vi "Main.vi"() -> ()   [LabVIEW 2017]
doc: "The myRIO Project template acquires acceleration data from the onboard accelerometer and displays the changes of acceleration values in a waveform chart."
uses:
  <vilib>/myRIO/Instrument Drivers/Onboard IO/DIO/typedefs/DIO Reference.ctl
  <vilib>/myRIO/Common/Instrument Driver Framework/Utilities/typedefs/myRIO Generic Hardware Reference.ctl
  <vilib>/myRIO/Common/Instrument Driver Framework/Utilities/typedefs/Hardware Version Enum.ctl
  <vilib>/myRIO/Common/Instrument Driver Framework/Utilities/typedefs/myRIO v1.0 Reference.ctl
  <vilib>/myRIO/Common/Instrument Driver Framework/Utilities/typedefs/Generic FPGA Reference.ctl
  <vilib>/myRIO/Common/Instrument Driver Framework/myRIO v1.0/DIO/typedefs/DIO Channels List.ctl
  <vilib>/myRIO/Common/Instrument Driver Framework/myRIO v1.0/DIO/typedefs/DIO Channels Enum.ctl
  <vilib>/userdefined/High Color/nirio_resource_hc.ctl
  <vilib>/Platform/TimedLoop/XDataNode/timing_clust.ctl
  <vilib>/Platform/TimedLoop/XDataNode/nitl_modes.ctl
  <vilib>/Platform/TimedLoop/XDataNode/wakeup.ctl
  <vilib>/myRIO/Instrument Drivers/Onboard IO/PWM/typedefs/PWM Reference.ctl
  <vilib>/myRIO/Common/Instrument Driver Framework/myRIO v1.0/PWM/typedefs/PWM Channels Enum.ctl
  <vilib>/myRIO/Instrument Drivers/Onboard IO/PWM/typedefs/PWM Configuration.ctl
  <vilib>/myRIO/Common/Instrument Driver Framework/myRIO v1.0/Encoder/typedefs/Encoder Signal Mode.ctl
  <vilib>/myRIO/Instrument Drivers/Onboard IO/Encoder/typedefs/Encoder Reference.ctl
  <vilib>/myRIO/Common/Instrument Driver Framework/myRIO v1.0/Encoder/typedefs/Encoder Channels Enum.ctl
  <vilib>/myRIO/Common/Instrument Driver Framework/myRIO v1.0/Encoder/typedefs/Encoder Configuration v1.0.ctl
  <vilib>/myRIO/Instrument Drivers/Onboard IO/AI/typedefs/AI Reference.ctl
  <vilib>/myRIO/Common/Instrument Driver Framework/myRIO v1.0/AI/typedefs/AI Channels List.ctl
  <vilib>/myRIO/Common/Instrument Driver Framework/myRIO v1.0/AI/typedefs/AI Channels Enum.ctl
  <vilib>/myRIO/Common/Instrument Driver Framework/Utilities/typedefs/Analog Scaling Constants List.ctl
  <vilib>/myRIO/Common/Instrument Driver Framework/Utilities/typedefs/Analog Scaling Constants.ctl
  <vilib>/myRIO/Common/Instrument Driver Framework/Utilities/vis/Is FPGA Ref Available.vi
  <vilib>/myRIO/Common/Instrument Driver Framework/myRIO v1.0/DIO/vis/myRIO v1.1 Open DIO.vi
  <vilib>/myRIO/Instrument Drivers/Onboard IO/DIO/vis/Write.vi
  <vilib>/myRIO/Common/Instrument Driver Framework/myRIO v1.0/PWM/vis/myRIO v1.1 Open PWM.vi
  <vilib>/myRIO/Instrument Drivers/Onboard IO/PWM/vis/Set Duty Cycle and Frequency.vi
  <vilib>/myRIO/Common/Instrument Driver Framework/myRIO v1.0/AI/vis/myRIO v1.1 Open AI.vi
  <vilib>/myRIO/Instrument Drivers/Onboard IO/AI/vis/Read.vi
  <vilib>/myRIO/Common/Instrument Driver Framework/myRIO v1.0/Encoder/vis/myRIO v1.1 Open Encoder.vi
  <vilib>/myRIO/Instrument Drivers/Onboard IO/Encoder/vis/Read.vi
  <vilib>/myRIO/Common/Instrument Driver Framework/Utilities/vis/Validate Channels.vi
  <vilib>/myRIO/Common/Instrument Driver Framework/myRIO v1.0/DIO/vis/myRIO v1.0 Reserve DIO.vi
  <vilib>/myRIO/Common/Instrument Driver Framework/myRIO v1.0/PWM/vis/myRIO v1.0 Reserve PWM.vi
  <vilib>/myRIO/Common/Instrument Driver Framework/myRIO v1.0/AI/vis/myRIO v1.0 Reserve AI.vi
  <vilib>/myRIO/Common/Instrument Driver Framework/myRIO v1.0/Encoder/vis/myRIO v1.0 Reserve Encoder.vi
  <vilib>/myRIO/Common/Instrument Driver Framework/myRIO v1.0/Resource Manager/vis/myRIO v1.0 Reserve Channel List.vi
  <vilib>/myRIO/Common/Instrument Driver Framework/myRIO v1.0/DIO/vis/myRIO v1.0 Build MUX Configuration DIO.vi
  <vilib>/myRIO/Common/Instrument Driver Framework/myRIO v1.0/PWM/vis/myRIO v1.0 Build MUX Configuration PWM.vi
  <vilib>/myRIO/Common/Instrument Driver Framework/myRIO v1.0/AI/vis/myRIO v1.0 Build MUX Configuration AI.vi
  <vilib>/myRIO/Common/Instrument Driver Framework/myRIO v1.0/Encoder/vis/myRIO v1.0 Build MUX Configuration Encoder.vi
  <vilib>/myRIO/Common/Instrument Driver Framework/myRIO v1.0/Resource Manager/vis/myRIO v1.0 Reserve Channel.vi
  <vilib>/myRIO/Common/Instrument Driver Framework/myRIO v1.0/Resource Manager/vis/myRIO v1.0 Unreserve Channel.vi
  <vilib>/myRIO/Common/Instrument Driver Framework/myRIO v1.0/Resource Manager/vis/myRIO v1.0 Create Configuration List.vi
  <vilib>/myRIO/Common/Instrument Driver Framework/myRIO v1.0/Resource Manager/vis/myRIO v1.0 Build Mutex Name.vi
  <vilib>/Utility/VariantDataType/GetNumericInfo.vi
  <vilib>/Utility/error.llb/Error Cluster From Error Code.vi
  <vilib>/myRIO/Common/Instrument Driver Framework/myRIO v1.0/myRIO v1.1 Open.vi
  <vilib>/myRIO/Common/Instrument Driver Framework/Utilities/vis/IO Manager.vi
  <vilib>/myRIO/Common/Instrument Driver Framework/Utilities/vis/Configuration Manager.vi
  <vilib>/myRIO/Common/Instrument Driver Framework/myRIO v1.0/Resource Manager/vis/myRIO v1.0 Configure IO.vi
  <vilib>/myRIO/Common/Instrument Driver Framework/myRIO v1.0/myRIO v1.0 Close.vi
  <vilib>/myRIO/Common/Instrument Driver Framework/myRIO v1.0/DIO/vis/myRIO v1.0 Write DIO.vi
  <vilib>/myRIO/Common/Instrument Driver Framework/myRIO v1.0/PWM/vis/myRIO v1.0 Write PWM.vi
  <vilib>/myRIO/Common/Instrument Driver Framework/myRIO v1.0/Encoder/vis/myRIO v1.0 Configure Encoder.vi
  <vilib>/myRIO/Common/Instrument Driver Framework/myRIO v1.0/Encoder/vis/myRIO v1.0 Read Encoder.vi
  <vilib>/myRIO/Common/Instrument Driver Framework/myRIO v1.0/AI/vis/myRIO v1.0 Get Scaling Constants AI.vi
  <vilib>/myRIO/Common/Instrument Driver Framework/myRIO v1.0/AI/vis/myRIO v1.0 Read AI.vi
  <vilib>/myRIO/Express VI/Onboard IO/DO/DO Express VI.xnode
  <vilib>/myRIO/Instrument Drivers/Onboard IO/DIO/vis/myRIO DIO Open.xnode
  <vilib>/myRIO/Express VI/Onboard IO/PWM/PWM Express VI.xnode
  <vilib>/myRIO/Instrument Drivers/Onboard IO/PWM/vis/myRIO PWM Open.xnode
  <vilib>/platform/TimedLoop/XDataNode/XDataNode.xnode
  <vilib>/myRIO/Express VI/Onboard IO/Encoder/Encoder Express VI.xnode
  <vilib>/myRIO/Instrument Drivers/Onboard IO/Encoder/vis/myRIO Encoder Open.xnode
  <vilib>/myRIO/Express VI/Onboard IO/AI/AI Express VI.xnode
  <vilib>/myRIO/Instrument Drivers/Onboard IO/AI/vis/myRIO AI Open.xnode
  <vilib>/myRIO/Instrument Drivers/Onboard IO/DIO/DIO.lvlib
  <vilib>/myRIO/Instrument Drivers/Onboard IO/PWM/PWM.lvlib
  <vilib>/myRIO/Instrument Drivers/Onboard IO/AI/AI.lvlib
  <vilib>/myRIO/Instrument Drivers/Onboard IO/Encoder/Encoder.lvlib
  <vilib>/Platform/TimedLoop/XDataNode/XDNodeRunTimeDep.lvlib
panel:
  in  "LIMin":dbl=15.0 min=0.0 step=0.1
  out "dt":dbl
  in  "Zerar Rede Neural":bool
  out "Aceleração da Ponta":dbl(graph)
  out "accp":dbl
  out "thpp":dbl
  out "thp":dbl
  out "Thetapp":cluster{"Thetapp":dbl, "thppD":dbl}(graph)
  out "Thetap":cluster{"Thetap":dbl, "thpD":dbl}(graph)
  out "Theta":cluster{"Theta":dbl, "thD":dbl}(graph)
  out "th":dbl
  in  "srpC":dbl=60.0 min=1.0 step=1.0
  in  "kIN":dbl=20.0 min=1.0 step=1.0
  in  "phiIN":dbl=15.0 step=0.1
  in  "apIN":dbl=1.8 min=0.0 step=0.1
  in  "Min":dbl=100.0 min=1.0 step=1.0
  in  "Funcionamento":bool
  in  "Lambda":dbl=15.0 min=0.0 max=10000.0 step=0.1
  in  "Tab Control":T1(tab)=enum."Controle Cossenoidal"
  in  "Posicao Angular":dbl(knob) min=-45.0 max=45.0 step=5.0 scale=45.0..-45.0
  in  "Amplitude":dbl(knob)=45.0 min=0.0 max=45.0 step=1.0 scale=0.0..45.0
  in  "Frequencia (Hz)":dbl(knob)=0.10000000000000002 min=0.0 max=3.0 step=0.1 scale=0.0..3.0
  in  "Amplitude":dbl(knob)=45.0 min=0.0 max=45.0 step=1.0 scale=0.0..45.0
  in  "Frequencia (Hz)":dbl(knob)=0.10000000000000002 min=0.0 max=3.0 step=0.1 scale=0.0..3.0
  in  "Período":dbl(knob)=2.5 min=1.5 max=10.0 step=0.5 scale=1.5..10.0
  in  "Reducao de vibração":bool=TRUE
  in  "Ciclo de Controle":bool
  out "th(°)":dbl
  in  "Zerar contador":bool
  in  "Ciclo de aquisição":bool
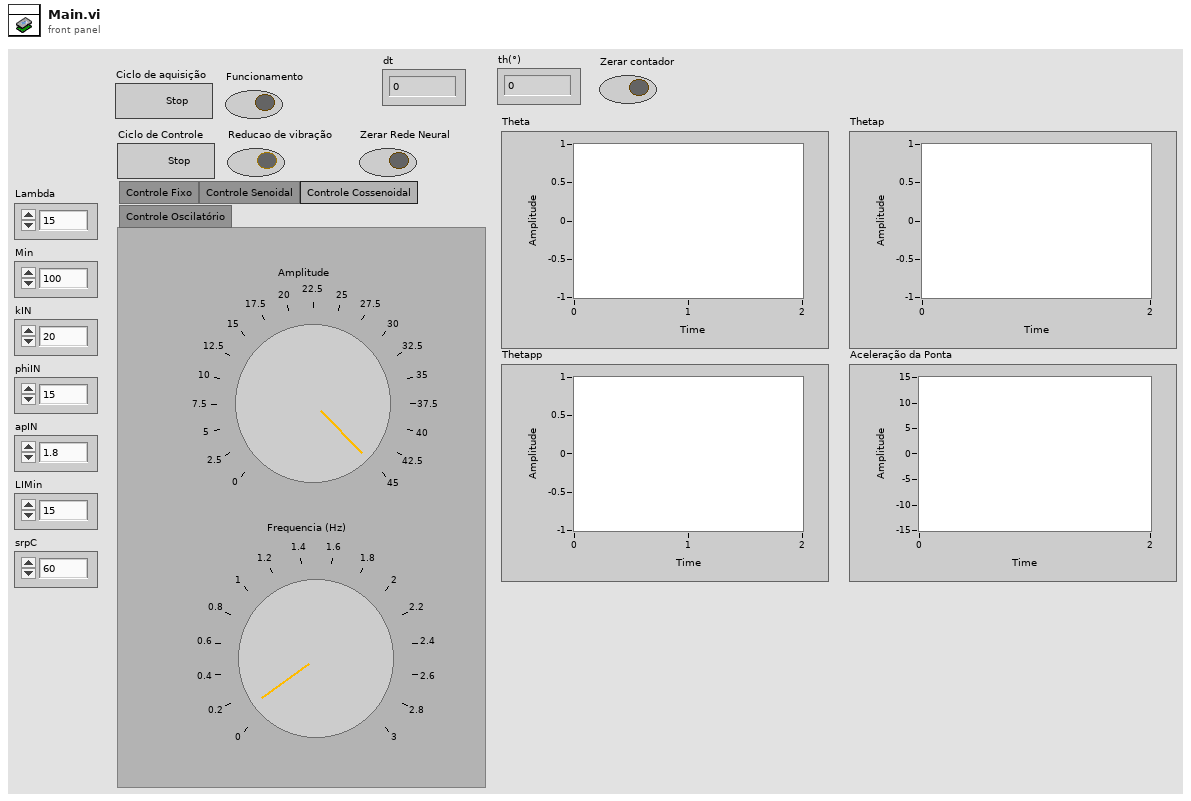
[diagram p1: front panel]
types:
  T1 = enum32{"Controle Fixo", "Controle Senoidal", "Controle Cossenoidal", "Controle Oscilatório"}
  T2 = typedef "DIO.lvlib/DIO Reference.ctl" = cluster{"myRIO Reference":T3, "DIO Channels List":T7}
  T3 = typedef "myRIO Generic Hardware Reference.ctl" = cluster{"myRIO Model":T4, "myRIO Hardware Reference":T5}
  T4 = typedef "Hardware Version Enum.ctl" = enum16{"Unknown", "myRIO-1900", "myRIO-1950", "roboRIO", "NI ELVIS RIO CM"}
  T5 = typedef "myRIO v1.0 Reference.ctl" = cluster{"Generic FPGA Reference":T6, "Allow multiple opens":bool}
  T6 = typedef "Generic FPGA Reference.ctl" = refnum<k20>
  T7 = typedef "DIO Channels List.ctl" = T8[]
  T8 = typedef "DIO Channels Enum.ctl" = enum16{"Not Connected", "C/DIO0", "C/DIO1", "C/DIO2", "C/DIO3", "C/DIO4", "C/DIO5", "C/DIO6", "C/DIO7", "A/DIO0", "A/DIO1", "A/DIO2", "A/DIO3", "A/DIO4", "A/DIO5", "A/DIO6", "A/DIO7", "A/DIO8", "A/DIO9", "A/DIO10", "A/DIO11", "A/DIO12", "A/DIO13", "A/DIO14", "A/DIO15", "B/DIO0", "B/DIO1", "B/DIO2", "B/DIO3", "B/DIO4", "B/DIO5", "B/DIO6", "B/DIO7", "B/DIO8", "B/DIO9", "B/DIO10", "B/DIO11", "B/DIO12", "B/DIO13", "B/DIO14", "B/DIO15", "LED0", "LED1", "LED2", "LED3", "Button0", "DIO/DIO0", "DIO/DIO1", "DIO/DIO2", "DIO/DIO3", "DIO/DIO4", "DIO/DIO5", "DIO/DIO6", "DIO/DIO7", "DIO/DIO8", "DIO/DIO9", "SPI/CS0", "SPI/CS1", "SPI/CS2", "SPI/CS3", "LED RADIO (Green)", "LED RADIO (Red)", "LED COMM (Green)", "LED COMM (Red)", "LED MODE (Green)", "LED MODE (Red)"}
  T9 = typedef "nirio_resource_hc.ctl" = tag
  T10 = typedef "XDNodeRunTimeDep.lvlib/timing_clust.ctl" = cluster{"Expected End [f-1]":u64, "Actual End [f-1]":u64, "Finished Late? [f-1]":bool, "Expected End [i-1]":u64, "Actual End [i-1]":u64, "Finished Late? [i-1]":bool, "Expected Start [i]":u64, "Actual Start [i]":u64, "Expected Start [f]":u64, "Actual Start [f]":u64, "Source Name":string, "Structure Name":string, "Period":i64, "Deadline":i64, "Offset":i64, "Start":i64, "Priority":i32, "Timeout":i32, "Mode":T11, "Wakeup Reason":T12, "Error":errorcluster, "Source Type":string, "Secondary Source Type":string, "Global End Time":u64, "Global Start Time":u64, "Frame Duration":u64, "Iteration Duration":u64, "Assigned CPU":i32, "I/O Scan Engine Mode":u32}
  T11 = typedef "XDNodeRunTimeDep.lvlib/nitl_modes.ctl" = enum32{"No Change", "Process missed periods, maintain original phase", "Discard missed periods, maintain original phase", "Process missed periods, ignore original phase", "Discard missed periods, ignore original phase"}
  T12 = typedef "XDNodeRunTimeDep.lvlib/wakeup.ctl" = enum32{"Normal", "Aborted", "Asynchronous wakeup", "Timing source error", "Timed loop error", "Timeout"}
  T13 = typedef "Encoder.lvlib/Encoder Reference.ctl" = cluster{"myRIO Reference":T3, "Encoder Channels Enum":T14}
  T14 = typedef "Encoder Channels Enum.ctl" = enum16{"Not Connected", "C/ENC0", "C/ENC1", "A/ENC", "B/ENC", "DIO/ENC0", "DIO/ENC1", "DIO/ENC2", "DIO/ENC3", "DIO/ENC4"}
  T15 = typedef "Encoder Signal Mode.ctl" = enum16{"Quadrature phase signal", "Step and direction signal"}
  T16 = typedef "AI.lvlib/AI Reference.ctl" = cluster{"myRIO Reference":T3, "AI Channels List":T17, "AI Scaling Constants List":T19}
  T17 = typedef "AI Channels List.ctl" = T18[]
  T18 = typedef "AI Channels Enum.ctl" = enum16{"Not Connected", "AudioIn/Left", "AudioIn/Right", "C/AI0", "C/AI1", "A/AI0", "A/AI1", "A/AI2", "A/AI3", "B/AI0", "B/AI1", "B/AI2", "B/AI3", "AI/AI0", "AI/AI1", "AI/AI2", "AI/AI3"}
  T19 = typedef "Analog Scaling Constants List.ctl" = T20[]
  T20 = typedef "Analog Scaling Constants.ctl" = cluster{"LSB Weight (Volts)":dbl, "Offset (Volts)":dbl, "Signed?":bool}
  T21 = typedef "PWM.lvlib/PWM Reference.ctl" = cluster{"myRIO Reference":T3, "PWM Channels Enum":T22, "PWM Configuration":T23}
  T22 = typedef "PWM Channels Enum.ctl" = enum16{"Not Connected", "C/PWM0", "C/PWM1", "A/PWM0", "A/PWM1", "A/PWM2", "B/PWM0", "B/PWM1", "B/PWM2", "PWM/PWM0", "PWM/PWM1", "PWM/PWM2", "PWM/PWM3", "PWM/PWM4", "PWM/PWM5", "PWM/PWM6", "PWM/PWM7", "PWM/PWM8", "PWM/PWM9"}
  T23 = typedef "PWM.lvlib/PWM Configuration.ctl" = cluster{"Frequency":dbl, "Duty Cycle":dbl}
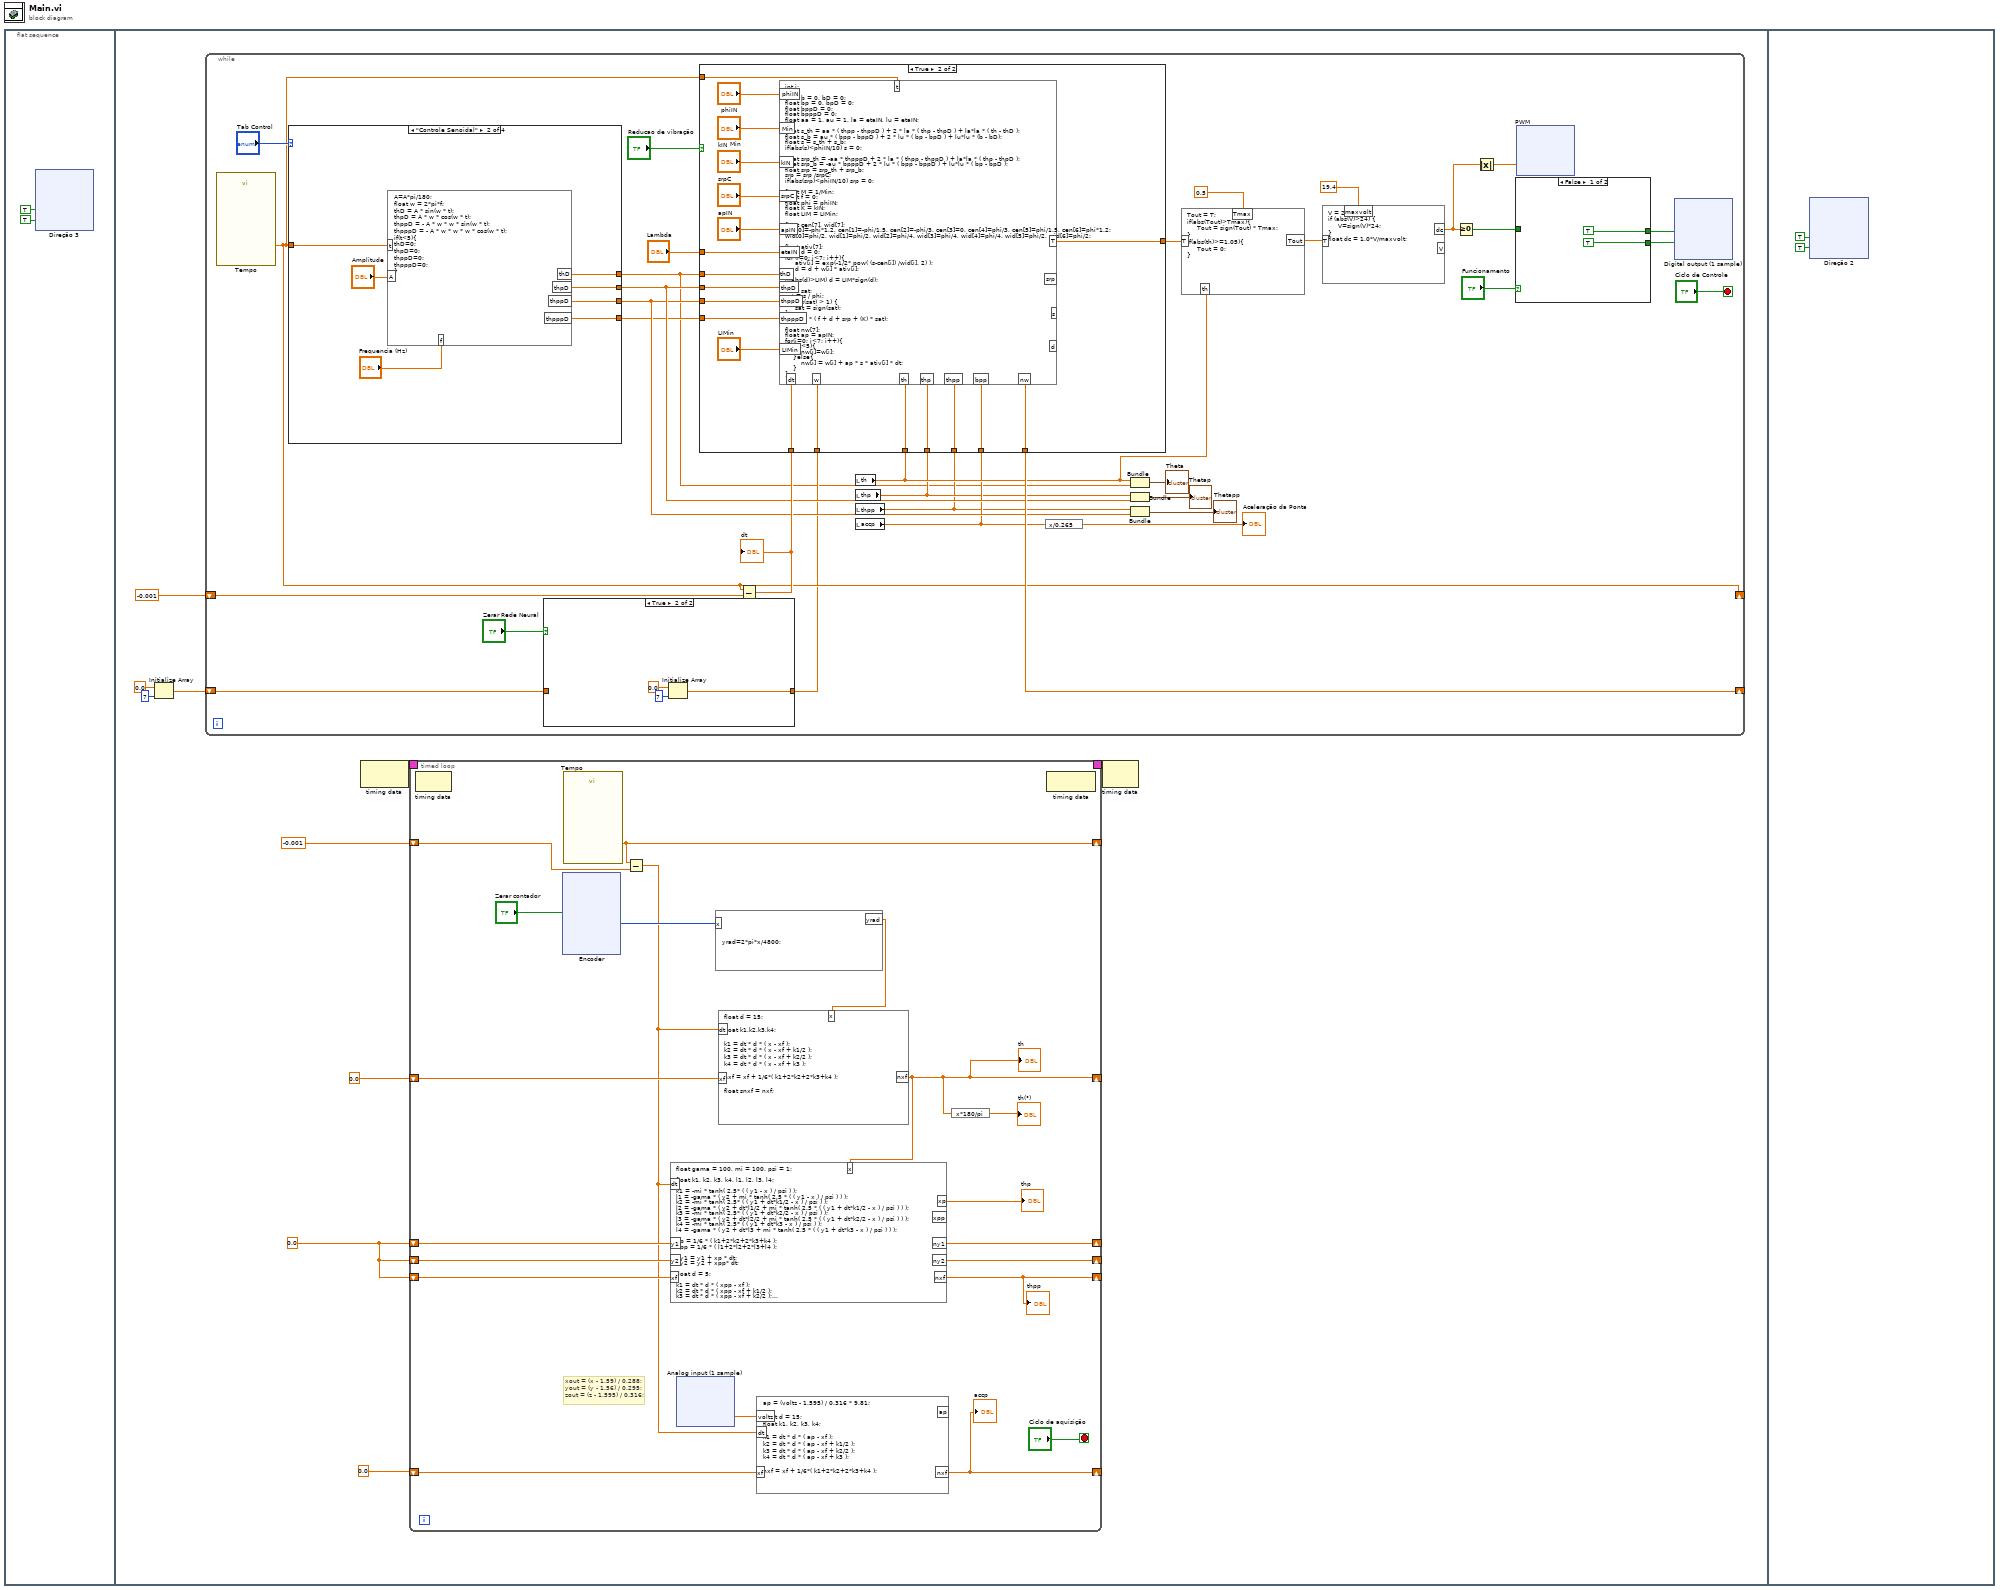
[diagram p0: block diagram]
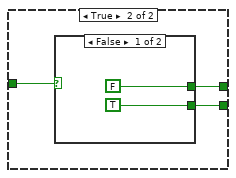
[diagram p2: hidden frame]
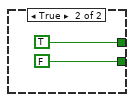
[diagram p3: hidden frame]
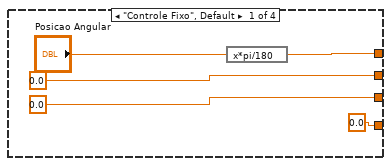
[diagram p4: hidden frame]
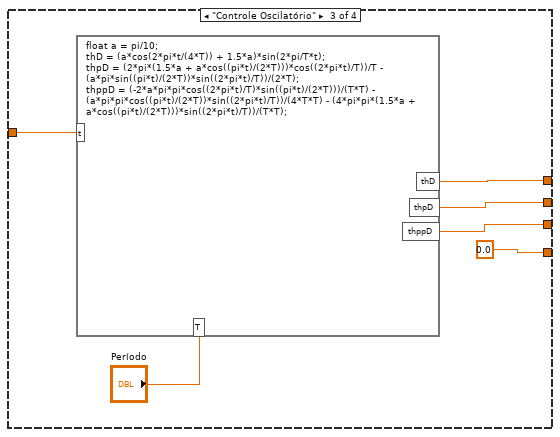
[diagram p5: hidden frame]
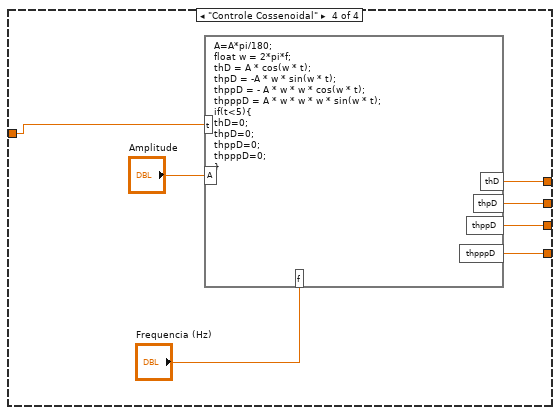
[diagram p6: hidden frame]
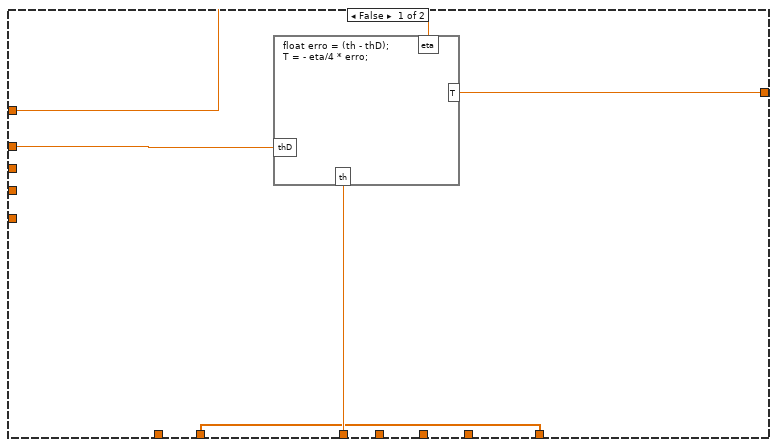
[diagram p7: hidden frame]
diagram:
  n1 = flat-sequence {
    frame #0 {
      n2 = xnode "Direção 3"("In1 (A/DIO8 (Pin 27))"=TRUE, "In2 (A/DIO9 (Pin 29))"=TRUE) -> ()  [unwired: 1 in, 1 out]
    }
    frame #1 {
      w45 = 0.0
      n3 = Initialize Array(0.0 ("element"), 7 ("dimension size")) -> (w43:dbl[])
      n4 = while {
        shift-right: [w181] -> _
        shift-left: w43 -> [w167]
        shift-right: [w159] -> _
        shift-left: -0.001 ("element") -> [w180]
        stop <- "Ciclo de Controle" stop-if-true
        n5 = call "Tempo"() -> ("Elapsed Time (s)"=w159:dbl)  [unwired: 12 in, 7 out]
        n6 = case shown="\"Controle Senoidal\"" "Tab Control" {
          tunnel: [w199 w208 w212 w218] -> w156
          tunnel: w159 -> [_ w207 w210 w219]
          tunnel: [0.0 w204 w213 w217] -> w173
          tunnel: [0.0 w203 w214 w216] -> w172
          tunnel: [0.0 ("thpppD") w202 0.0 ("thpppD") w215] -> w161
          frame "Controle Fixo", Default {
            n7 = expression code="x*pi/180"("Posicao Angular") -> (w199:dbl)
          }
          frame "Controle Senoidal" {
            n8 = formula code="A=A*pi/180;\nfloat w = 2*pi*f;\nthD = A * sin(w * t);\nthpD = A * w * cos(w * t);\nthppD = - A * w * w * sin(w * t);\nthpppD = - A * w * w * w * cos(w * t);\nif(t<5){\nthD=0;\nthpD=0;\nthppD=0;\nthpppD=0;\n}"("t"=w207, "A"="Amplitude", "f"="Frequencia (Hz)") -> ("thD"=w208:dbl, "thpD"=w204:dbl, "thppD"=w203:dbl, "thpppD"=w202:dbl)
          }
          frame "Controle Oscilatório" {
            n9 = formula code="float a = pi/10;\nthD = (a*cos(2*pi*t/(4*T)) + 1.5*a)*sin(2*pi/T*t);\nthpD = (2*pi*(1.5*a + a*cos((pi*t)/(2*T)))*cos((2*pi*t)/T))/T - (a*pi*sin((pi*t)/(2*T))*sin((2*pi*t)/T))/(2*T);\nthppD = (-2*a*pi*pi*cos((2*pi*t)/T)*sin((pi*t)/(2*T)))/(T*T) - (a*pi*pi*cos((pi*t)/(2*T))*sin((2*pi*t)/T))/(4*T*T) - (4*pi*pi*(1.5*a + a*cos((pi*t)/(2*T)))*sin((2*pi*t)/T))/(T*T);"("t"=w210, "T"="Período") -> ("thD"=w212:dbl, "thpD"=w213:dbl, "thppD"=w214:dbl)
          }
          frame "Controle Cossenoidal" {
            n10 = formula code="A=A*pi/180;\nfloat w = 2*pi*f;\nthD = A * cos(w * t);\nthpD = -A * w * sin(w * t);\nthppD = - A * w * w * cos(w * t);\nthpppD = A * w * w * w * sin(w * t);\nif(t<5){\nthD=0;\nthpD=0;\nthppD=0;\nthpppD=0;\n}"("t"=w219, "A"="Amplitude", "f"="Frequencia (Hz)") -> ("thD"=w218:dbl, "thpD"=w217:dbl, "thppD"=w216:dbl, "thpppD"=w215:dbl)
          }
        }
        n11 = case shown="True" "Zerar Rede Neural" {
          tunnel: [w318 w319] -> w157
          tunnel: w167 -> [w318 _]
          frame False {
          }
          frame True {
            n12 = Initialize Array(0.0 ("element"), 7 ("dimension size")) -> (w319:dbl[])
          }
        }
        n13 = Subtract(x=w159, y=w180) -> (x-y=w179:dbl)
        "dt" <- w179
        n14 = local read "th"() -> (w166:dbl)
        n15 = local read "thp"() -> (w163:dbl)
        n16 = local read "thpp"() -> (w160:dbl)
        n17 = local read "accp"() -> (w165:dbl)
        n18 = case shown="True" "Reducao de vibração" {
          tunnel: w156 -> [w226 w238]
          tunnel: [w225 w246] -> w155
          tunnel: "Lambda" -> [w224 w245]
          tunnel: [w222 w235] -> w181
          tunnel: w179 -> [_ w244]
          tunnel: w173 -> [_ w237]
          tunnel: w172 -> [_ w236]
          tunnel: w165 -> [_ w234]
          tunnel: w160 -> [_ w233]
          tunnel: w163 -> [_ w232]
          tunnel: w166 -> [w223 w231]
          tunnel: w157 -> [w222 w230]
          tunnel: w161 -> [_ w229]
          tunnel: w159 -> [_ w228]
          frame False {
            n19 = formula code="float erro = (th - thD);\nT = - eta/4 * erro;"("thD"=w226, "th"=w223, "eta"=w224) -> ("T"=w225:dbl)
          }
          frame True {
            n20 = formula code="int i;\n\nfloat b = 0, bD = 0;\nfloat bp = 0, bpD = 0;\nfloat bppD = 0;\nfloat bpppD = 0;\nfloat aa = 1, au = 1, la = etaIN, lu = etaIN;\n\nfloat s_th = aa * ( thpp - thppD ) + 2 * la * ( thp - thpD ) + la*la * ( th - thD );\nfloat s_b = au * ( bpp - bppD ) + 2 * lu * ( bp - bpD ) + lu*lu * (b - bD);\nfloat s = s_th + s_b;\nif(abs(s)<phiIN/10) s = 0;\n\nfloat srp_th = -aa * thpppD + 2 * la * ( thpp - thppD ) + la*la * ( thp - thpD );\nfloat srp_b = -au * bpppD + 2 * lu * ( bpp - bppD ) + lu*lu * ( bp - bpD );\nfloat srp = srp_th + srp_b;\nsrp = srp /srpC;\nif(abs(srp)<phiIN/10) srp = 0;\n\nfloat M = 1/Min;\nfloat f = 0;\nfloat phi = phiIN;\nfloat K = kIN;\nfloat LIM = LIMin;\n\nfloat cen[7], wid[7];\ncen[0]=-phi*1.2, cen[1]=-phi/1.5, cen[2]=-phi/3, cen[3]=0, cen[4]=phi/3, cen[5]=phi/1.5, cen[6]=phi*1.2;\nwid[0]=phi/2, wid[1]=phi/2, wid[2]=phi/4, wid[3]=phi/4, wid[4]=phi/4, wid[5]=phi/2, wid[6]=phi/2;\n\nfloat ativ[7];\nfloat d = 0;\nfor (i=0; i<7; i++){\n     ativ[i] = exp(-1/2* pow( (s-cen[i]) /wid[i], 2) );\n     d = d + w[i] * ativ[i];\n}\nif(abs(d)>LIM) d = LIM*sign(d);\n\nfloat sat;\nsat = s / phi;\nif (abs(sat) > 1) {\n     sat = sign(sat);\n}\nT = - M * ( f + d + srp + (K) * sat);\n\nfloat nw[7];\nfloat ap = apIN;\nfor(i=0; i<7; i++){\n    if(t<5){\n        nw[i]=w[i];\n    }else{\n        nw[i] = w[i] + ap * s * ativ[i] * dt;\n    }\n}"("thD"=w238, "th"=w231, "thp"=w232, "thpp"=w233, "bpp"=w234, "etaIN"=w245, "w"=w230, "dt"=w244, "Min"="Min", "apIN"="apIN", "phiIN"="phiIN", "kIN"="kIN", "srpC"="srpC", "thpD"=w237, "thppD"=w236, "t"=w228, "thpppD"=w229, "LIMin"="LIMin") -> ("T"=w246:dbl, "nw"=w235:dbl[])  [unwired: 3 out]
          }
        }
        n21 = expression code="x/0.265"(w165) -> (→"Aceleração da Ponta":dbl)
        n22 = Bundle("th"=w166, "thD"=w156) -> (→"Theta":cluster{"th":dbl, "thD":dbl})  [unwired: 1 in]
        n23 = Bundle("thp"=w163, "thpD"=w173) -> (→"Thetap":cluster{"thp":dbl, "thpD":dbl})  [unwired: 1 in]
        n24 = Bundle("thpp"=w160, "thppD"=w172) -> (→"Thetapp":cluster{"thpp":dbl, "thppD":dbl})  [unwired: 1 in]
        n25 = formula code="Tout = T;\nif(abs(Tout)>Tmax){\n     Tout = sign(Tout) * Tmax;\n}\nif(abs(th)>=1.05){\n     Tout = 0;\n}"("Tmax"=0.5 ("input variable"), "T"=w155, "th"=w166) -> ("Tout"=w164:dbl)
        n26 = formula code="V = 24/3*T;\nif (abs(V)>24) {\n     V=sign(V)*24;\n}\nfloat dc = 1.0*V/maxvolt;"("maxvolt"=19.4 ("input variable"), "T"=w164) -> ("dc"=w158:dbl)  [unwired: 1 out]
        n27 = Greater Or Equal To 0?(x=w158) -> (x >= 0?=w178:bool)
        n28 = Absolute Value(x=w158) -> (abs(x)=w186:dbl)
        n29 = case shown="False" "Funcionamento" {
          tunnel: w178 -> [_ w192]
          tunnel: [TRUE w191] -> w177
          tunnel: [TRUE w190] -> w176
          frame False {
          }
          frame True {
            n30 = case shown="False" w192 {
              tunnel: [FALSE TRUE] -> w191
              tunnel: [TRUE FALSE] -> w190
              frame False {
              }
              frame True {
              }
            }
          }
        }
        n31 = xnode "PWM"("Duty Cycle"=w186) -> ()  [unwired: 1 in, 1 out]
        n32 = xnode "Digital output (1 sample)"("In1 (A/DIO8 (Pin 27))"=w177, "In2 (A/DIO9 (Pin 29))"=w176) -> ()  [unwired: 1 in, 1 out]
      }
      n33 = node-c288() -> (w48:T10)  [unwired: 1 in]
      n34 = timed-loop {
        shift-right: [w62] -> _
        shift-left: -0.001 -> [w64]
        shift-right: [w60] -> _
        shift-left: w45 -> [w66]
        shift-right: [w65] -> _
        shift-left: w45 -> [w59]
        shift-right: [w50] -> _
        shift-left: w45 -> [w63]
        timing: w48 -> [_]
        timing-out: [_] -> w47
        shift-right: [w52] -> _
        shift-left: 0.0 -> [w57]
        shift-right: [w49] -> _
        shift-left: 0.0 ("nxf") -> [w54]
        stop <- "Ciclo de aquisição" stop-if-true
        # "xout = (x - 1.59) / 0.288;\nyout = (y - 1.56) / 0.295;\nzout = (z - 1.595) / 0.316;"
        n35 = node-c288() -> ()  [unwired: 1 in, 1 out]
        n36 = xnode "Encoder"("Reset Counter"="Zerar contador") -> ("Counter Value"=w67:i32)  [unwired: 1 in, 3 out]
        n37 = call "Tempo"() -> ("Elapsed Time (s)"=w62:dbl)  [unwired: 12 in, 7 out]
        n38 = Subtract(x=w62, y=w64) -> (x-y=w53:dbl)
        n39 = xnode "Analog input (1 sample)"() -> ("Acc (A/AI2 (Pin 7))"=w61:dbl)  [unwired: 1 in, 1 out]
        n40 = formula code="yrad=2*pi*x/4800;"("x"=w67) -> ("yrad"=w56:dbl)
        n41 = formula code="float d = 15;\n\nfloat k1,k2,k3,k4;\n\nk1 = dt * d * ( x - xf );\nk2 = dt * d * ( x - xf + k1/2 );\nk3 = dt * d * ( x - xf + k2/2 );\nk4 = dt * d * ( x - xf + k3 );\n\nnxf = xf + 1/6*( k1+2*k2+2*k3+k4 );\n\nfloat snxf = nxf;"("x"=w56, "xf"=w57, "dt"=w53) -> ("nxf"=w52:dbl)
        "th" <- w52
        n42 = formula code="float gama = 100, mi = 100, psi = 1;\n\nfloat k1, k2, k3, k4, l1, l2, l3, l4;\n\nk1 = -mi * tanh( 2.5* ( ( y1 - x ) / psi ) );\nl1 = -gama * ( y2 + mi * tanh( 2.5 * ( ( y1 - x ) / psi ) ) );\nk2 = -mi * tanh( 2.5* ( ( y1 + dt*k1/2 - x ) / psi ) );\nl2 = -gama * ( y2 + dt*l1/2 + mi * tanh( 2.5 * ( ( y1 + dt*k1/2 - x ) / psi ) ) );\nk3 = -mi * tanh( 2.5* ( ( y1 + dt*k2/2 - x ) / psi ) );\nl3 = -gama * ( y2 + dt*l2/2 + mi * tanh( 2.5 * ( ( y1 + dt*k2/2 - x ) / psi ) ) );\nk4 = -mi * tanh( 2.5* ( ( y1 + dt*k3 - x ) / psi ) );\nl4 = -gama * ( y2 + dt*l3 + mi * tanh( 2.5 * ( ( y1 + dt*k3 - x ) / psi ) ) );\n\nxp = 1/6 * ( k1+2*k2+2*k3+k4 );\nxpp = 1/6 * ( l1+2*l2+2*l3+l4 );\n\nny1 = y1 + xp * dt;\nny2 = y2 + xpp* dt;\n\nfloat d = 5;\n\nk1 = dt * d * ( xpp - xf );\nk2 = dt * d * ( xpp - xf + k1/2 );\nk3 = dt * d * ( xpp - xf + k2/2 );\nk4 = dt * d * ( xpp - xf + k3 );\n\nnxf = xf + 1/6*( k1+2*k2+2*k3+k4 );"("y1"=w59, "y2"=w66, "x"=w52, "dt"=w53, "xf"=w63) -> ("ny1"=w65:dbl, "ny2"=w60:dbl, "xp"=→"thp":dbl, "nxf"=w50:dbl)  [unwired: 1 out]
        "thpp" <- w50
        n43 = formula code="ap = (voltz - 1.595) / 0.316 * 9.81;\n\nfloat d = 15;\nfloat k1, k2, k3, k4;\n\nk1 = dt * d * ( ap - xf );\nk2 = dt * d * ( ap - xf + k1/2 );\nk3 = dt * d * ( ap - xf + k2/2 );\nk4 = dt * d * ( ap - xf + k3 );\n\nnxf = xf + 1/6*( k1+2*k2+2*k3+k4 );"("voltz"=w61, "dt"=w53, "xf"=w54) -> ("nxf"=w49:dbl)  [unwired: 1 out]
        "accp" <- w49
        n44 = expression code="x*180/pi"(w52) -> (→"th(°)":dbl)
        n45 = node-c288() -> ()  [unwired: 1 in, 1 out]
      }
      n46 = node-c288(w47) -> ()  [unwired: 1 out]
    }
    frame #2 {
      n47 = xnode "Direção 2"("In1 (A/DIO8 (Pin 27))"=TRUE, "In2 (A/DIO9 (Pin 29))"=TRUE) -> ()  [unwired: 1 in, 1 out]
    }
  }
